vi "SetGetContTimeModeParams.vi"() -> ()   [LabVIEW 2017]
uses:
  AT901 API/Structures/Struct ContinuousTimeModeData.ctl
  AT901 API/TypeDefinitions/ES_RegionType.ctl
panel:
  in  "ContinuousTimeModeData 2":T1={"TimeSeparation"=100, "NumberOfPoints"=0, "UseRegion"=FALSE, "ES_RegionType"=enum."ES_RT_Sphere"}
  out "ContinuousTimeModeData":T1={"TimeSeparation"=0, "NumberOfPoints"=0, "UseRegion"=TRUE, "ES_RegionType"=enum."ES_RT_Sphere"}
  out "error out":errorcluster
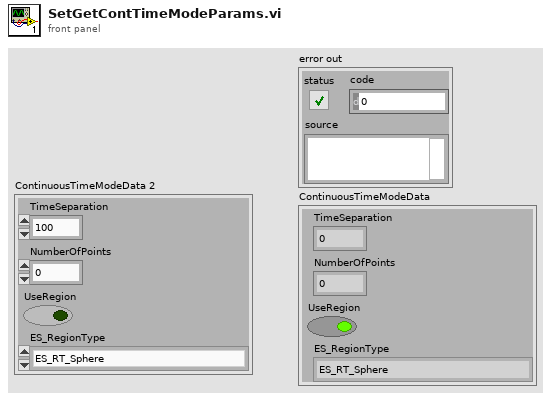
[diagram p1: front panel]
types:
  T1 = typedef "Struct ContinuousTimeModeData.ctl" = cluster{"TimeSeparation":u32, "NumberOfPoints":u32, "UseRegion":bool, "ES_RegionType":T2}
  T2 = typedef "ES_RegionType.ctl" = enum32{"ES_RT_Sphere", "ES_RT_Box"}
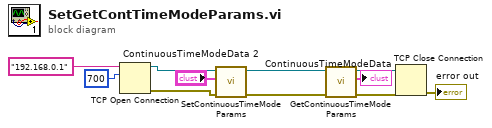
[diagram p0: block diagram]
diagram:
  n1 = TCP Open Connection(address="192.168.0.1", remote port or service name=u16 700) -> (connection ID=w8:refnum<k5>, error out=w7:errorcluster)  [unwired: 3 in]
  n2 = call "SetContinuousTimeModeParams.vi"("error in (no error)"=w7, "ContinuousTimeModeData"="ContinuousTimeModeData 2", "TCP Network Connection in"=w8) -> ("error out"=w5:errorcluster, "TCP Network Connection out"=w6:refnum<k5>)  [unwired: 5 in, 2 out]
  n3 = call "GetContinuousTimeModeParams.vi"("error in (no error)"=w5, "TCP Network Connection in"=w6) -> ("error out"=w4:errorcluster, "ContinuousTimeModeData"=→"ContinuousTimeModeData":T1, "TCP Network Connection out"=w3:refnum<k5>)  [unwired: 5 in, 2 out]
  n4 = TCP Close Connection(connection ID=w3, error in (no error)=w4) -> (error out=→"error out":errorcluster)  [unwired: 1 in, 1 out]
